vi "Create Data Server Thread.vi"(7 "period (100 ms)":u32=100 format="%d ms", 8 "error in (no error)":errorcluster, 10 "Framework Configuration":refnum<class "Framework Configuration.lvclass">, 11 "Buffers":T1) -> (0 "error out":errorcluster, 2 "Interface":refnum<class "Plugin Interface.lvclass">, 3 "Data Server Thread out":refnum<class "Data Server Thread.lvclass">)   [LabVIEW 2019, in "DSF Core.lvlib" / "Data Server Thread.lvclass"]
uses:
  Data Server Thread.lvclass
  C:/Dev/GitHub/niveristand-data-sharing-framework-custom-device/Core/Classes/Thread/Thread.lvclass
  Framework.ctl
  Buffers/Buffers.lvclass
  Status/Status Pointer.lvclass
  Plugin.ctl
  Group.ctl
  Transfer/Transfer.lvclass
  Interface/Plugin/Plugin Interface.lvclass
  Configuration/Core/Framework/Framework Configuration.lvclass
  Thread Settings.ctl
  Data Server Thread.lvclass/Data Server Thread.ctl
  Thread.lvclass
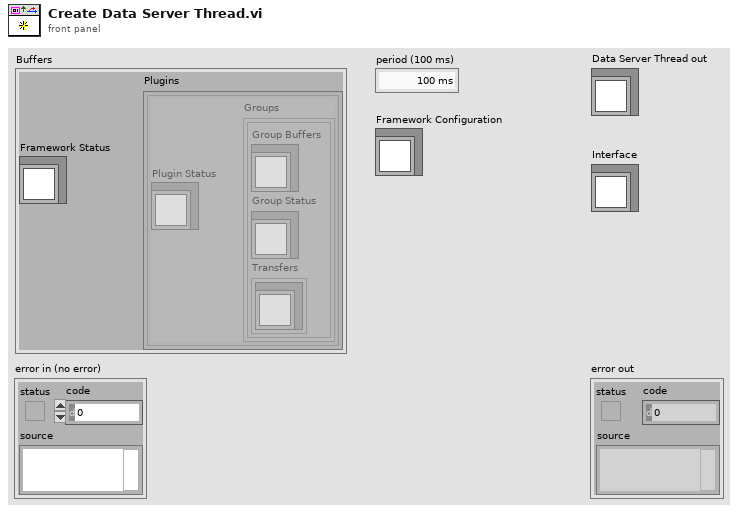
[diagram p1: front panel]
types:
  T1 = typedef "DSF Core.lvlib/Data Server Thread.lvclass/Framework.ctl" = cluster{"Framework Status":refnum<class "Status Pointer.lvclass">, "Plugins":T2[]}
  T2 = typedef "DSF Core.lvlib/Data Server Thread.lvclass/Plugin.ctl" = cluster{"Plugin Status":refnum<class "Status Pointer.lvclass">, "Groups":T3[]}
  T3 = typedef "DSF Core.lvlib/Data Server Thread.lvclass/Group.ctl" = cluster{"Group Buffers":refnum<class "Buffers.lvclass">, "Group Status":refnum<class "Status Pointer.lvclass">, "Transfers":refnum<class "Transfer.lvclass">[]}
  T4 = enum16{"big-endian, network order", "native, host order", "little-endian"}
  T5 = typedef "DSF Core.lvlib/Thread.lvclass/Thread Settings.ctl" = cluster{"Priority":u16, "Processor":i32}
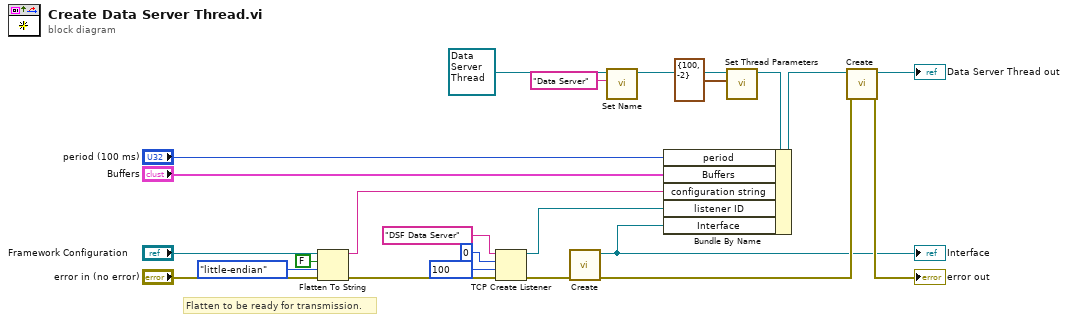
[diagram p0: block diagram]
diagram:
  # "Flatten to be ready for transmission."
  n1 = Flatten To String(anything="Framework Configuration", prepend array or string size? (T)=FALSE, byte order (0:big-endian, network order)=T4."little-endian", error in (no error)="error in (no error)") -> (data string=w4:string, error out=w6:errorcluster)  [unwired: 1 out]
  n2 = TCP Create Listener(8:w6, 9:100 ("timeout ms (25000)"), 10:u16 0 ("port"), 11:"DSF Data Server" ("service name")) -> (0:w15:errorcluster, 3:w5:refnum<k5>)  [unwired: 1 in, 1 out]
  n3 = call "Create.vi"("error in (no error)"=w15) -> ("error out"=w14:errorcluster, "Plugin Interface"=w13:refnum<class "Plugin Interface.lvclass">)  [unwired: 9 in]
  "Interface" <- w13
  n4 = call "Set Name.vi"("name"="Data Server", "Thread in"=refnum<class "Data Server Thread.lvclass"> refnum ("Data Server Thread out")) -> ("Thread out"=w10:refnum<class "Data Server Thread.lvclass">)  [unwired: 9 in]
  n5 = call "Set Thread Parameters.vi"("thread settings"=T5 {"Priority"=100, "Processor"=-2}, "Thread in"=w10) -> ("Thread out"=w9:refnum<class "Data Server Thread.lvclass">)  [unwired: 9 in]
  n6 = Bundle By Name(cluster=w9, "period"="period (100 ms)", "Buffers"="Buffers", "configuration string"=w4, "listener ID"=w5, "Interface"=w13) -> (w21:refnum<class "Data Server Thread.lvclass">)
  n7 = call-dynamic "Create.vi"("error in (no error)"=w14, "Thread in"=w21) -> ("error out"=→"error out":errorcluster, "Thread out"=→"Data Server Thread out":refnum<class "Data Server Thread.lvclass">)  [unwired: 8 in]
